vi "View Insert VI.vi"(8 "error in (no error)":errorcluster, 9 "ViewMap":map{string, T1}(c390), 10 "Name":string, 11 "TabControl in":refnum<vi>) -> (0 "error out":errorcluster, 3 "TabControl in 2":refnum<vi>)   [LabVIEW 2020, in "MDI ViewManager.lvlib"]
uses:
  MDI ViewManager.lvlib
  Typedef/Update View.ctl
  <vilib>/Utility/miscctls.llb/LVBoundsTypeDef.ctl
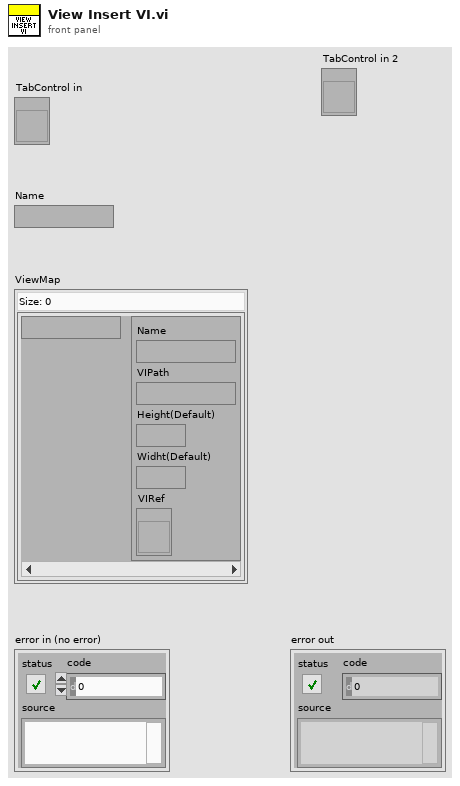
[diagram p1: front panel]
types:
  T1 = typedef "MDI ViewManager.lvlib/Update View.ctl" = cluster{"Name":string, "VIPath":path, "Height(Default)":u32, "Widht(Default)":u32, "VIRef":refnum<vi>}
  T2 = typedef "LVBoundsTypeDef.ctl" = cluster{"Width":u32, "Height":u32}
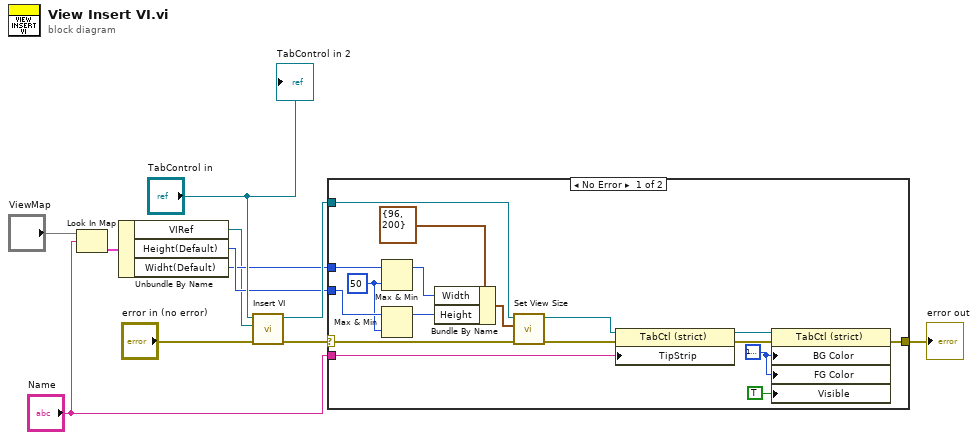
[diagram p0: block diagram]
diagram:
  n1 = Look In Map(map="ViewMap", key="Name") -> (value=w3:T1)  [unwired: 1 in, 1 out]
  n2 = Unbundle By Name(w3) -> ("VIRef"=w6:refnum<vi>, "Height(Default)"=w8:u32, "Widht(Default)"=w7:u32)
  n3 = call "Insert VI.vi"("error in (no error)"="error in (no error)", "VIRef"=w6, "TabControl in"="TabControl in") -> ("error out"=w9:errorcluster, "TabControl out"=w10:refnum<vi>)  [unwired: 7 in]
  n4 = case shown="No Error" w9 {
    selector: w9 -> [w22 w29]
    tunnel: "Name" -> [w25 _]
    tunnel: w10 -> [w24 _]
    tunnel: w8 -> [w28 _]
    tunnel: w7 -> [w27 _]
    tunnel: [w13 w29] -> w1
    frame No Error {
      w16 = u32 16777216 ("Colors:BG Color")
      w26 = u32 50 ("y")
      n5 = Max & Min(x=w27, y=w26) -> (max(x,y)=w18:u32)  [unwired: 1 out]
      n6 = Max & Min(x=w28, y=w26) -> (max(x,y)=w17:u32)  [unwired: 1 out]
      n7 = Bundle By Name(cluster=T2 {"Width"=96, "Height"=200} ("TabDimension"), "Width"=w18, "Height"=w17) -> (w19:T2)
      n8 = call "Set View Size.vi"("error in (no error)"=w22, "TabDimension"=w19, "TabControlRef in"=w24) -> ("error out"=w21:errorcluster, "TabControlRef out"=w23:refnum<vi>)  [unwired: 7 in]
      n9 = property class="TabCtl (strict)"(reference=w23, error in=w21, "TipStrip"=w25) -> (reference out=w15:refnum<vi>, error out=w14:errorcluster)
      n10 = property class="TabCtl (strict)"(reference=w15, error in=w14, "BG Color"=w16, "FG Color"=w16, "Visible"=TRUE) -> (error out=w13:errorcluster)  [unwired: 1 out]
    }
    frame Error {
    }
  }
  "error out" <- w1
  "TabControl in 2" <- "TabControl in"
